vi "set_initial_value.vi"(6 "item":T1={"name"="", "data type"=1, "access level"=1, "description"=""} {"data type" items=["Boolean"=1, "SByte"=2, "Byte"=3, "Int16"=4, "UInt16"=5, "Int32"=6, "UInt32"=7, "Int64"=8, "UInt64"=9, "Float"=10, "Double"=11, "String"=12, "DateTime"=13, "ByteString"=15, "Array of Boolean"=101, "Array of SByte"=102, "Array of Byte"=103, "Array of Int16"=104, "Array of UInt16"=105, "Array of Int32"=106, "Array of UInt32"=107, "Array of Int64"=108, "Array of UInt64"=109, "Array of Float"=110, "Array of Double"=111, "Array of String"=112, "Array of DateTime"=113, "Array of ByteString"=115]; "access level" items=["read-only"=1, "write-only"=2, "read/write"=3]}, 8 "Error In":errorcluster, 9 "value string":string, 10 "node path":string, 11 "OPC UA server refnum in":refnum<k21>) -> (0 "Error Out":errorcluster, 2 "node path (dup)":string, 3 "OPC UA server refnum out":refnum<k21>)   [LabVIEW 2013, in "CreateOPCUAServerAuto.lvlib"]
uses:
  CreateOPCUAServerAuto.lvlib
  <vilib>/OPCUA/server/Write Bool.vi
  <vilib>/OPCUA/server/Write SByte.vi
  <vilib>/OPCUA/server/Write Byte.vi
  <vilib>/OPCUA/server/Write Int16.vi
  <vilib>/OPCUA/server/Write UInt16.vi
  <vilib>/OPCUA/server/Write Int32.vi
  <vilib>/OPCUA/server/Write UInt32.vi
  <vilib>/OPCUA/server/Write Int64.vi
  <vilib>/OPCUA/server/Write UInt64.vi
  <vilib>/OPCUA/server/Write Float.vi
  <vilib>/OPCUA/server/Write Double.vi
  <vilib>/OPCUA/server/Write String.vi
  <vilib>/OPCUA/server/Write Date Time.vi
  <vilib>/OPCUA/server/Write Byte String.vi
  <vilib>/OPCUA/server/Write Bool Array.vi
  <vilib>/OPCUA/server/Write SByte Array.vi
  <vilib>/OPCUA/server/Write Byte Array.vi
  <vilib>/OPCUA/server/Write Int16 Array.vi
  <vilib>/OPCUA/server/Write UInt16 Array.vi
  <vilib>/OPCUA/server/Write Int32 Array.vi
  <vilib>/OPCUA/server/Write UInt32 Array.vi
  <vilib>/OPCUA/server/Write Int64 Array.vi
  <vilib>/OPCUA/server/Write UInt64 Array.vi
  <vilib>/OPCUA/server/Write Float Array.vi
  <vilib>/OPCUA/server/Write Double Array.vi
  <vilib>/OPCUA/server/Write String Array.vi
  <vilib>/OPCUA/server/Write Date Time Array.vi
  <vilib>/OPCUA/server/Write Byte String Array.vi
  <vilib>/OPCUA/NI OPC UA Server.lvlib
panel:
  out "value string 2":string
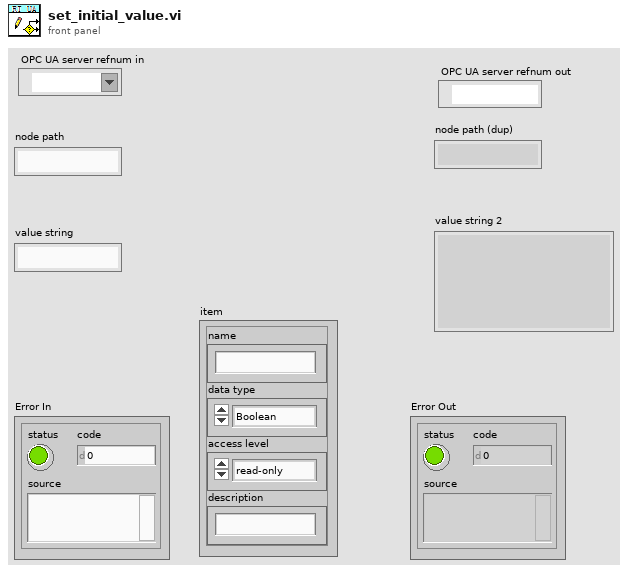
[diagram p1: front panel]
types:
  T1 = cluster{"name":string, "data type":u16, "access level":u16, "description":string}
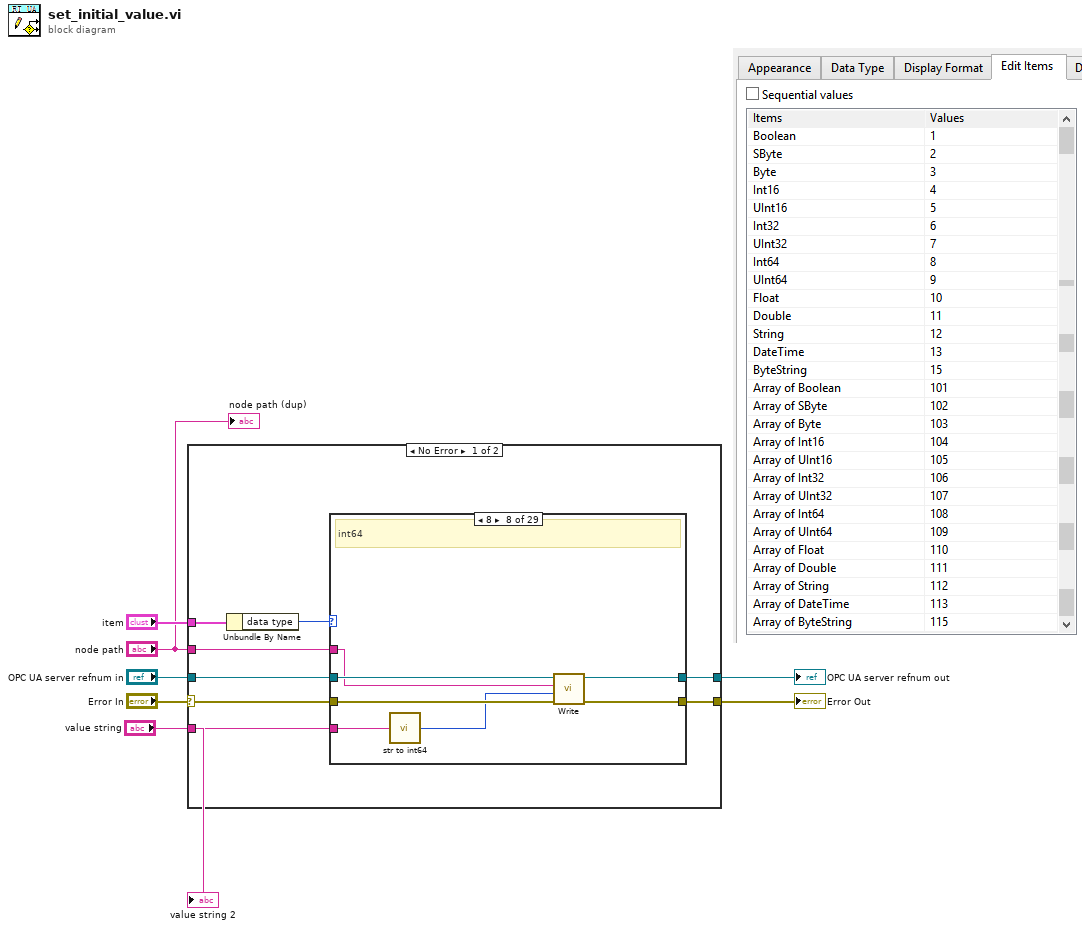
[diagram p0: block diagram]
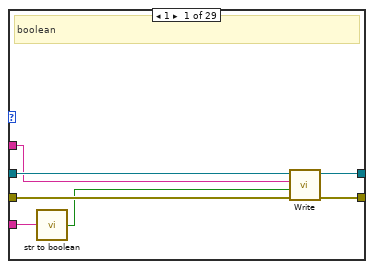
[diagram p2: hidden frame]
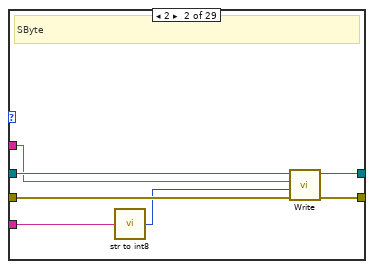
[diagram p3: hidden frame]
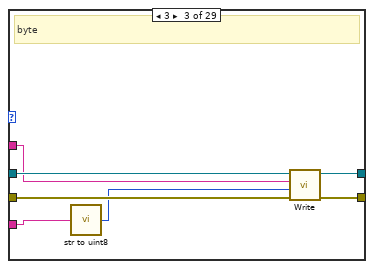
[diagram p4: hidden frame]
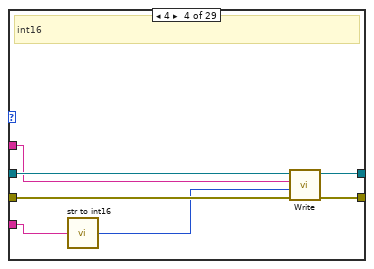
[diagram p5: hidden frame]
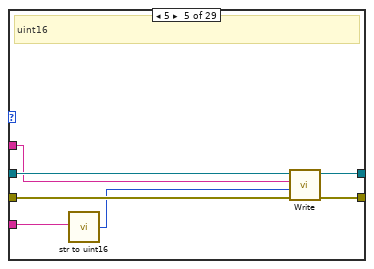
[diagram p6: hidden frame]
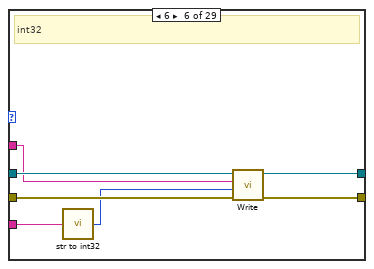
[diagram p7: hidden frame]
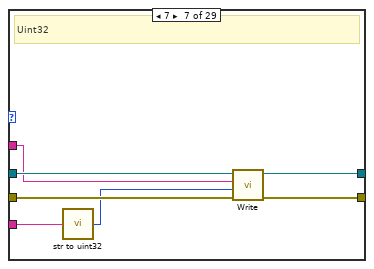
[diagram p8: hidden frame]
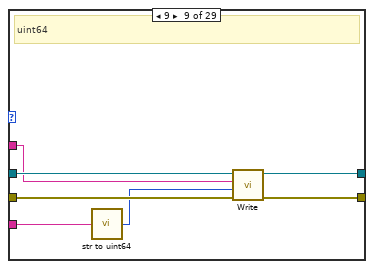
[diagram p9: hidden frame]
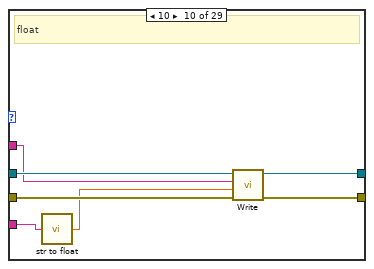
[diagram p10: hidden frame]
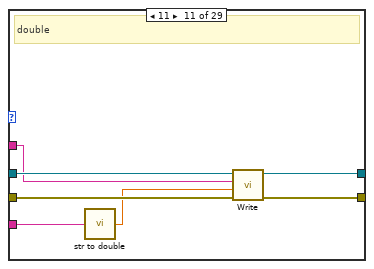
[diagram p11: hidden frame]
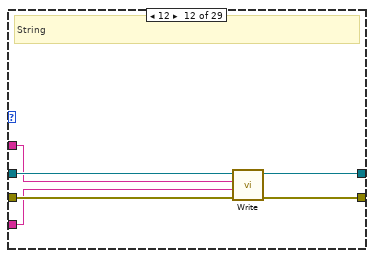
[diagram p12: hidden frame]
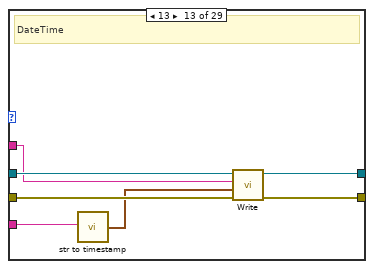
[diagram p13: hidden frame]
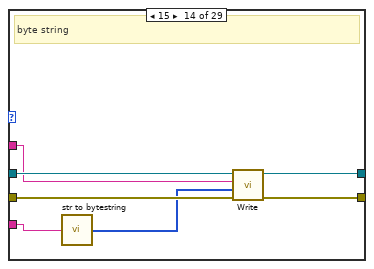
[diagram p14: hidden frame]
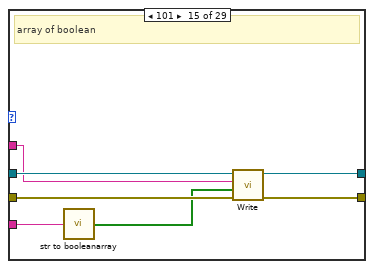
[diagram p15: hidden frame]
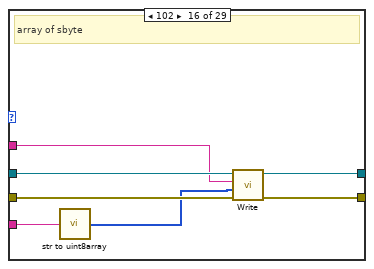
[diagram p16: hidden frame]
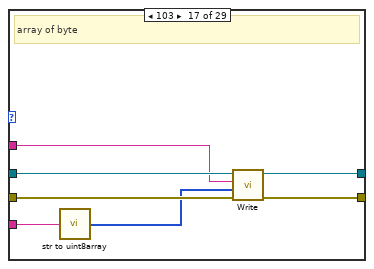
[diagram p17: hidden frame]
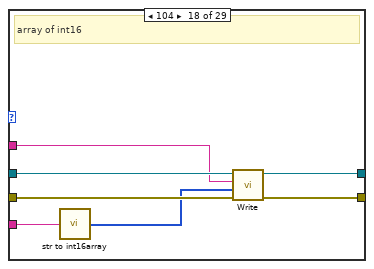
[diagram p18: hidden frame]
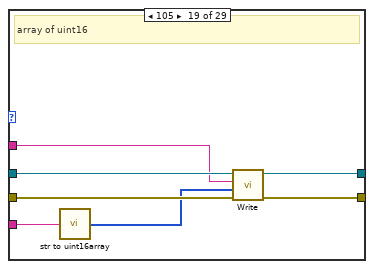
[diagram p19: hidden frame]
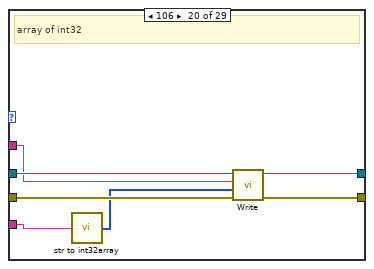
[diagram p20: hidden frame]
diagram:
  n1 = case shown="No Error" "Error In" {
    selector: "Error In" -> [w15 w218]
    tunnel: [w10 w218] -> w7
    tunnel: "OPC UA server refnum in" -> [w14 w217]
    tunnel: [w9 w217] -> w4
    tunnel: "item" -> [w13 _]
    tunnel: "node path" -> [w12 _]
    tunnel: "value string" -> [w8 _]
    frame No Error {
      n2 = Unbundle By Name(w13) -> ("data type"=w11:u16)
      n3 = case shown="8" w11 {
        tunnel: w15 -> [w22 w29 w36 w43 w50 w54 w61 w68 w75 w82 w89 w95 w102 w109 w116 w123 w130 w137 w144 w151 w158 w165 w172 w179 w186 w193 w200 w207 w215]
        tunnel: w14 -> [w19 w26 w33 w40 w47 w55 w62 w69 w76 w83 w90 w96 w103 w110 w117 w124 w131 w138 w145 w152 w159 w166 w173 w180 w187 w194 w201 w208 w216]
        tunnel: w12 -> [w18 w25 w32 w39 w46 w53 w60 w67 w74 w81 w88 w94 w101 w108 w115 w122 w129 w136 w143 w150 w157 w164 w171 w178 w185 w192 w199 w206 _]
        tunnel: [w21 w28 w35 w42 w49 w56 w63 w70 w77 w84 w91 w97 w104 w111 w118 w125 w132 w139 w146 w153 w160 w167 w174 w181 w188 w195 w202 w209 w211] -> w10
        tunnel: [w20 w27 w34 w41 w48 w57 w64 w71 w78 w85 w92 w98 w105 w112 w119 w126 w133 w140 w147 w154 w161 w168 w175 w182 w189 w196 w203 w210 w216] -> w9
        tunnel: w8 -> [w17 w24 w30 w38 w45 w52 w59 w66 w73 w80 w87 w93 w100 w107 w114 w120 w128 w135 w142 w149 w156 w163 w170 w177 w184 w191 w198 w205 _]
        frame 1 {
          # "boolean"
          n4 = call "str to boolean.vi"("String"=w17) -> ("Boolean"=w16:bool)  [unwired: 6 in]
          n5 = call-poly <vilib>:"Write.vi"("error in (no error)"=w22, "value"=w16, "node path"=w18, "OPC UA server refnum in"=w19) -> ("error out"=w21:errorcluster, "OPC UA server refnum out"=w20:refnum<k21>)  [unwired: 6 in]
        }
        frame 2 {
          # "SByte"
          n6 = call "str to int8.vi"("String"=w24) -> ("int8"=w23:i8)  [unwired: 6 in]
          n7 = call-poly <vilib>:"Write.vi"("error in (no error)"=w29, "value"=w23, "node path"=w25, "OPC UA server refnum in"=w26) -> ("error out"=w28:errorcluster, "OPC UA server refnum out"=w27:refnum<k21>)  [unwired: 6 in]
        }
        frame 3 {
          # "byte"
          n8 = call "str to uint8.vi"("String"=w30) -> ("uint8"=w31:u8)  [unwired: 6 in]
          n9 = call-poly <vilib>:"Write.vi"("error in (no error)"=w36, "value"=w31, "node path"=w32, "OPC UA server refnum in"=w33) -> ("error out"=w35:errorcluster, "OPC UA server refnum out"=w34:refnum<k21>)  [unwired: 6 in]
        }
        frame 4 {
          # "int16"
          n10 = call "str to int16.vi"("String"=w38) -> ("int16"=w37:i16)  [unwired: 6 in]
          n11 = call-poly <vilib>:"Write.vi"("error in (no error)"=w43, "value"=w37, "node path"=w39, "OPC UA server refnum in"=w40) -> ("error out"=w42:errorcluster, "OPC UA server refnum out"=w41:refnum<k21>)  [unwired: 6 in]
        }
        frame 5 {
          # "uint16"
          n12 = call "str to uint16.vi"("String"=w45) -> ("uint16"=w44:u16)  [unwired: 6 in]
          n13 = call-poly <vilib>:"Write.vi"("error in (no error)"=w50, "value"=w44, "node path"=w46, "OPC UA server refnum in"=w47) -> ("error out"=w49:errorcluster, "OPC UA server refnum out"=w48:refnum<k21>)  [unwired: 6 in]
        }
        frame 6 {
          # "int32"
          n14 = call "str to int32.vi"("String"=w52) -> ("int32"=w51:i32)  [unwired: 6 in]
          n15 = call-poly <vilib>:"Write.vi"("error in (no error)"=w54, "value"=w51, "node path"=w53, "OPC UA server refnum in"=w55) -> ("error out"=w56:errorcluster, "OPC UA server refnum out"=w57:refnum<k21>)  [unwired: 6 in]
        }
        frame 7 {
          # "Uint32"
          n16 = call "str to uint32.vi"("String"=w59) -> ("uint32"=w58:u32)  [unwired: 6 in]
          n17 = call-poly <vilib>:"Write.vi"("error in (no error)"=w61, "value"=w58, "node path"=w60, "OPC UA server refnum in"=w62) -> ("error out"=w63:errorcluster, "OPC UA server refnum out"=w64:refnum<k21>)  [unwired: 6 in]
        }
        frame 8 {
          # "int64"
          n18 = call "str to int64.vi"("String"=w66) -> ("int64"=w65:i64)  [unwired: 6 in]
          n19 = call-poly <vilib>:"Write.vi"("error in (no error)"=w68, "value"=w65, "node path"=w67, "OPC UA server refnum in"=w69) -> ("error out"=w70:errorcluster, "OPC UA server refnum out"=w71:refnum<k21>)  [unwired: 6 in]
        }
        frame 9 {
          # "uint64"
          n20 = call "str to uint64.vi"("String"=w73) -> ("uint64"=w72:u64)  [unwired: 6 in]
          n21 = call-poly <vilib>:"Write.vi"("error in (no error)"=w75, "value"=w72, "node path"=w74, "OPC UA server refnum in"=w76) -> ("error out"=w77:errorcluster, "OPC UA server refnum out"=w78:refnum<k21>)  [unwired: 6 in]
        }
        frame 10 {
          # "float"
          n22 = call "str to float.vi"("String"=w80) -> ("float"=w79:sgl)  [unwired: 6 in]
          n23 = call-poly <vilib>:"Write.vi"("error in (no error)"=w82, "value"=w79, "node path"=w81, "OPC UA server refnum in"=w83) -> ("error out"=w84:errorcluster, "OPC UA server refnum out"=w85:refnum<k21>)  [unwired: 6 in]
        }
        frame 11 {
          # "double"
          n24 = call "str to double.vi"("String"=w87) -> ("double"=w86:dbl)  [unwired: 6 in]
          n25 = call-poly <vilib>:"Write.vi"("error in (no error)"=w89, "value"=w86, "node path"=w88, "OPC UA server refnum in"=w90) -> ("error out"=w91:errorcluster, "OPC UA server refnum out"=w92:refnum<k21>)  [unwired: 6 in]
        }
        frame 12 {
          # "String"
          n26 = call-poly <vilib>:"Write.vi"("error in (no error)"=w95, "value"=w93, "node path"=w94, "OPC UA server refnum in"=w96) -> ("error out"=w97:errorcluster, "OPC UA server refnum out"=w98:refnum<k21>)  [unwired: 6 in]
        }
        frame 13 {
          # "DateTime"
          n27 = call "str to timestamp.vi"("date/time string"=w100) -> ("Resulting Time Stamp"=w99:timestamp)
          n28 = call-poly <vilib>:"Write.vi"("error in (no error)"=w102, "value"=w99, "node path"=w101, "OPC UA server refnum in"=w103) -> ("error out"=w104:errorcluster, "OPC UA server refnum out"=w105:refnum<k21>)  [unwired: 6 in]
        }
        frame 15 {
          # "byte string"
          n29 = call "str to bytestring.vi"("String"=w107) -> ("value"=w106:u8[])  [unwired: 6 in]
          n30 = call-poly <vilib>:"Write.vi"("error in (no error)"=w109, "value"=w106, "node path"=w108, "OPC UA server refnum in"=w110) -> ("error out"=w111:errorcluster, "OPC UA server refnum out"=w112:refnum<k21>)  [unwired: 6 in]
        }
        frame 101 {
          # "array of boolean"
          n31 = call "str to booleanarray.vi"("String"=w114) -> ("boolean array"=w113:bool[])  [unwired: 6 in]
          n32 = call-poly <vilib>:"Write.vi"("error in (no error)"=w116, "value"=w113, "node path"=w115, "OPC UA server refnum in"=w117) -> ("error out"=w118:errorcluster, "OPC UA server refnum out"=w119:refnum<k21>)  [unwired: 6 in]
        }
        frame 102 {
          # "array of sbyte"
          n33 = call "str to uint8array.vi"("String"=w120) -> ("uint8 array"=w121:u8[])  [unwired: 6 in]
          n34 = call-poly <vilib>:"Write.vi"("error in (no error)"=w123, "value"=w121, "node path"=w122, "OPC UA server refnum in"=w124) -> ("error out"=w125:errorcluster, "OPC UA server refnum out"=w126:refnum<k21>)  [unwired: 6 in]
        }
        frame 103 {
          # "array of byte"
          n35 = call "str to uint8array.vi"("String"=w128) -> ("uint8 array"=w127:u8[])  [unwired: 6 in]
          n36 = call-poly <vilib>:"Write.vi"("error in (no error)"=w130, "value"=w127, "node path"=w129, "OPC UA server refnum in"=w131) -> ("error out"=w132:errorcluster, "OPC UA server refnum out"=w133:refnum<k21>)  [unwired: 6 in]
        }
        frame 104 {
          # "array of int16"
          n37 = call "str to int16array.vi"("String"=w135) -> ("int16 array"=w134:i16[])  [unwired: 6 in]
          n38 = call-poly <vilib>:"Write.vi"("error in (no error)"=w137, "value"=w134, "node path"=w136, "OPC UA server refnum in"=w138) -> ("error out"=w139:errorcluster, "OPC UA server refnum out"=w140:refnum<k21>)  [unwired: 6 in]
        }
        frame 105 {
          # "array of uint16"
          n39 = call "str to uint16array.vi"("String"=w142) -> ("uint16 array"=w141:u16[])  [unwired: 6 in]
          n40 = call-poly <vilib>:"Write.vi"("error in (no error)"=w144, "value"=w141, "node path"=w143, "OPC UA server refnum in"=w145) -> ("error out"=w146:errorcluster, "OPC UA server refnum out"=w147:refnum<k21>)  [unwired: 6 in]
        }
        frame 106 {
          # "array of int32"
          n41 = call "str to int32array.vi"("String"=w149) -> ("int32 array"=w148:i32[])  [unwired: 6 in]
          n42 = call-poly <vilib>:"Write.vi"("error in (no error)"=w151, "value"=w148, "node path"=w150, "OPC UA server refnum in"=w152) -> ("error out"=w153:errorcluster, "OPC UA server refnum out"=w154:refnum<k21>)  [unwired: 6 in]
        }
        frame 107 {
          # "array of uint32"
          n43 = call "str to uint32array.vi"("String"=w156) -> ("uint32 array"=w155:u32[])  [unwired: 6 in]
          n44 = call-poly <vilib>:"Write.vi"("error in (no error)"=w158, "value"=w155, "node path"=w157, "OPC UA server refnum in"=w159) -> ("error out"=w160:errorcluster, "OPC UA server refnum out"=w161:refnum<k21>)  [unwired: 6 in]
        }
        frame 108 {
          # "array of int64"
          n45 = call "str to int64array.vi"("String"=w163) -> ("int64 array"=w162:i64[])  [unwired: 6 in]
          n46 = call-poly <vilib>:"Write.vi"("error in (no error)"=w165, "value"=w162, "node path"=w164, "OPC UA server refnum in"=w166) -> ("error out"=w167:errorcluster, "OPC UA server refnum out"=w168:refnum<k21>)  [unwired: 6 in]
        }
        frame 109 {
          # "array of uint64"
          n47 = call "str to uint64array.vi"("String"=w170) -> ("uint64 array"=w169:u64[])  [unwired: 6 in]
          n48 = call-poly <vilib>:"Write.vi"("error in (no error)"=w172, "value"=w169, "node path"=w171, "OPC UA server refnum in"=w173) -> ("error out"=w174:errorcluster, "OPC UA server refnum out"=w175:refnum<k21>)  [unwired: 6 in]
        }
        frame 110 {
          # "array of float"
          n49 = call "str to floatarray.vi"("String"=w177) -> ("float array"=w176:sgl[])  [unwired: 6 in]
          n50 = call-poly <vilib>:"Write.vi"("error in (no error)"=w179, "value"=w176, "node path"=w178, "OPC UA server refnum in"=w180) -> ("error out"=w181:errorcluster, "OPC UA server refnum out"=w182:refnum<k21>)  [unwired: 6 in]
        }
        frame 111 {
          # "array of double"
          n51 = call "str to doublearray.vi"("String"=w184) -> ("double array"=w183:dbl[])  [unwired: 6 in]
          n52 = call-poly <vilib>:"Write.vi"("error in (no error)"=w186, "value"=w183, "node path"=w185, "OPC UA server refnum in"=w187) -> ("error out"=w188:errorcluster, "OPC UA server refnum out"=w189:refnum<k21>)  [unwired: 6 in]
        }
        frame 112 {
          # "array of string"
          n53 = call "str to strarray.vi"("String"=w191) -> ("str array"=w190:string[])  [unwired: 6 in]
          n54 = call-poly <vilib>:"Write.vi"("error in (no error)"=w193, "value"=w190, "node path"=w192, "OPC UA server refnum in"=w194) -> ("error out"=w195:errorcluster, "OPC UA server refnum out"=w196:refnum<k21>)  [unwired: 6 in]
        }
        frame 113 {
          # "array of datetime"
          n55 = call "str to datetimearray.vi"("String"=w198) -> ("timestamp array"=w197:timestamp[])  [unwired: 6 in]
          n56 = call-poly <vilib>:"Write.vi"("error in (no error)"=w200, "value"=w197, "node path"=w199, "OPC UA server refnum in"=w201) -> ("error out"=w202:errorcluster, "OPC UA server refnum out"=w203:refnum<k21>)  [unwired: 6 in]
        }
        frame 115 {
          # "array of bytestring"
          n57 = call "str to bytestringarray.vi"("String"=w205) -> ("bytestring array"=w204:u8[][])  [unwired: 6 in]
          n58 = call-poly <vilib>:"Write.vi"("error in (no error)"=w207, "value"=w204, "node path"=w206, "OPC UA server refnum in"=w208) -> ("error out"=w209:errorcluster, "OPC UA server refnum out"=w210:refnum<k21>)  [unwired: 6 in]
        }
        frame Default {
          n59 = Bundle By Name(cluster=w215, "status"=TRUE, "code"=-1, "source"="not supported data type") -> (w211:errorcluster)
        }
      }
    }
    frame Error {
    }
  }
  "Error Out" <- w7
  "OPC UA server refnum out" <- w4
  "node path (dup)" <- "node path"
  "value string 2" <- "value string"
